vi "normalize_vector.vi"(1 "Numeric":dbl, 2 "vector":cluster{"x":dbl, "y":dbl}) -> (0 "output":cluster{"x":dbl, "y":dbl})   [LabVIEW 2023]
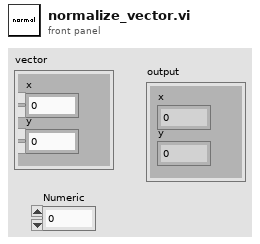
[diagram p1: front panel]
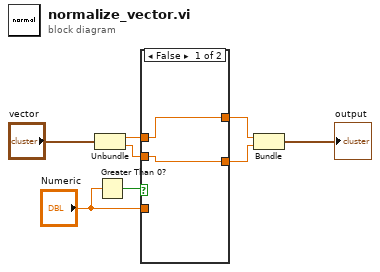
[diagram p0: block diagram]
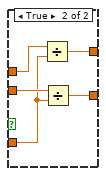
[diagram p2: hidden frame]
diagram:
  n1 = Unbundle("vector") -> ("x"=w7:dbl, "y"=w6:dbl)
  n2 = Greater Than 0?(x="Numeric") -> (x > 0?=w2:bool)
  n3 = case shown="False" w2 {
    tunnel: w7 -> [w10 w15]
    tunnel: w6 -> [w9 w14]
    tunnel: [w10 w13] -> w5
    tunnel: [w9 w12] -> w4
    tunnel: "Numeric" -> [_ w11]
    frame False {
    }
    frame True {
      n4 = Divide(x=w15, y=w11) -> (x/y=w13:dbl)
      n5 = Divide(x=w14, y=w11) -> (x/y=w12:dbl)
    }
  }
  n6 = Bundle("x"=w5, "y"=w4) -> (→"output":cluster{"x":dbl, "y":dbl})  [unwired: 1 in]
